vi "Draw Aimpoint.vi"(5 "Robot Y":dbl, 7 "Robot X":dbl, 11 "new picture in":picture) -> (3 "out":picture)   [LabVIEW 2013]
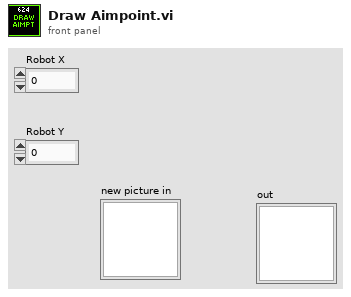
[diagram p1: front panel]
types:
  T1 = cluster{"Width":u16, "Style":enum32{"Solid", "Dash", "Dot", "DashDot", "DashDotDot"}}
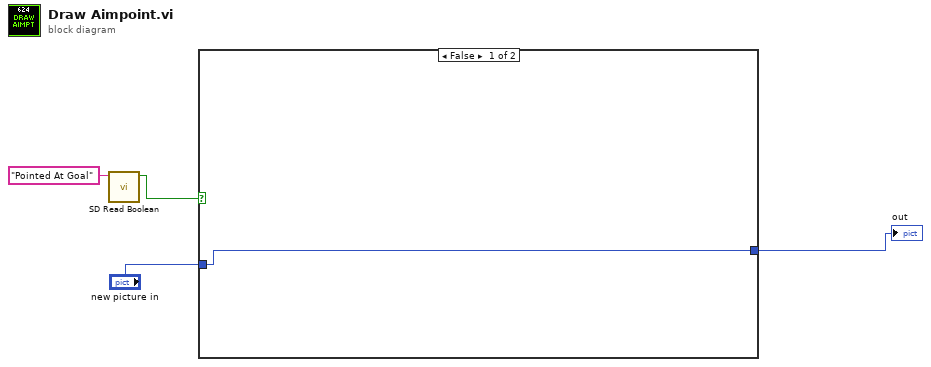
[diagram p0: block diagram]
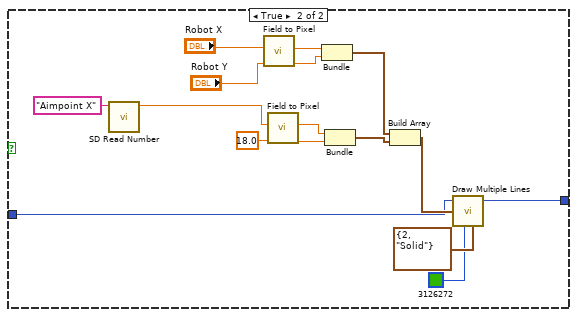
[diagram p2: hidden frame]
diagram:
  n1 = call <vilib>:"SD Read Boolean.vi"("Name"="Pointed At Goal") -> ("Boolean"=w1:bool)  [unwired: 8 in, 2 out]
  n2 = case shown="False" w1 {
    tunnel: "new picture in" -> [w5 w9]
    tunnel: [w5 w8] -> w3
    frame False {
    }
    frame True {
      n3 = call <vilib>:"SD Read Number.vi"("Name"="Aimpoint X") -> ("Numeric"=w18:dbl)  [unwired: 8 in, 2 out]
      n4 = call "Field to Pixel.vi"("Field Coordinate Y"="Robot Y", "Field Coordinate X"="Robot X") -> ("Pixel Y"=w15:dbl, "Pixel X"=w16:dbl)  [unwired: 8 in]
      n5 = call "Field to Pixel.vi"("Field Coordinate Y"=18.0, "Field Coordinate X"=w18) -> ("Pixel Y"=w13:dbl, "Pixel X"=w14:dbl)  [unwired: 8 in]
      n6 = Bundle("Pixel X"=w16, "Pixel Y"=w15) -> (w11:cluster{"Pixel X":dbl, "Pixel Y":dbl})  [unwired: 1 in]
      n7 = Bundle("Pixel X"=w14, "Pixel Y"=w13) -> (w12:cluster{"Pixel X":dbl, "Pixel Y":dbl})  [unwired: 1 in]
      n8 = Build Array(w11, w12) -> (w10:cluster{"Pixel X":dbl, "Pixel Y":dbl}[])
      n9 = call <vilib>:"Draw Multiple Lines.vi"("picture"=w9, "line endpoints"=w10, "color(black)"=u32 3126272, "pen"=T1 {"Width"=2, "Style"=enum."Solid"}) -> ("new picture"=w8:picture)  [unwired: 5 in]
    }
  }
  "out" <- w3
